vi "SSFG_sharp.vi"() -> ()   [LabVIEW 2014]
uses:
  SSFG_States.ctl
  <vilib>/Utility/error.llb/DialogType.ctl
  <vilib>/DAQmx/read.llb/DAQmx Read (Analog Wfm 1Chan NSamp).vi
  <vilib>/DAQmx/write.llb/DAQmx Write (Analog Wfm 1Chan NSamp).vi
  <vilib>/DAQmx/create/channels.llb/DAQmx Create Channel (AO-Voltage-Basic).vi
  <vilib>/DAQmx/create/channels.llb/DAQmx Create Channel (AI-Voltage-Basic).vi
  <vilib>/DAQmx/configure/timing.llb/DAQmx Timing (Sample Clock).vi
  <vilib>/DAQmx/miscellaneous.llb/DAQmx Fill In Error Info.vi
  <vilib>/measure/mascope.llb/Cycle Average and RMS 1 chan.vi
  <resource>/objmgr/daqmx.rc
  <vilib>/measure/NI_MABase.lvlib
  <vilib>/measure/NI_MAPro.lvlib
panel:
  in  "Physical Channel 2":tag="Dev1/ai0" caption="Physical Channel"
  in  "Sample Rate":dbl=10000.0 caption="Sample Rate (Hz)" format="%0.2f"
  out "Measurement":waveform(dbl)(graph)
  in  "stop 2":bool caption="stop"
  in  "Samples to Read":i32=1000
  out "cycle RMS":dbl format="%.2g"
  out "Numeric":i32
  out "Buffer Space":u32
  out "Iterations":i32
  in  "Attenuation":dbl
  in  "Number of Samples/Cycle":dbl
  out "Generation":waveform(dbl)(graph)
  in  "stop":bool
  in  "Power Signal Parameters":T1={"Waveform Type"=0, "Amplitude"=1.0, "Frequency"=17.0} {"Frequency" format="%0.2p"; "Waveform Type" items=["Sine Wave", "Triangle Wave", "Square Wave", "Sawtooth Wave"]}
  out "Flicker":bool
  out "Swell":bool
  out "Sag":bool
  in  "Stop":bool
  in  "Update Rate":dbl=1000.0 format="%0.2f"
  in  "Generation":tag
  in  "Flicker":T2
  in  "Swell":cluster{"Swell_Time (sec)":dbl, "Swell":bool}
  in  "Sag":cluster{"Sag_Time (sec)":dbl, "Sag":bool}
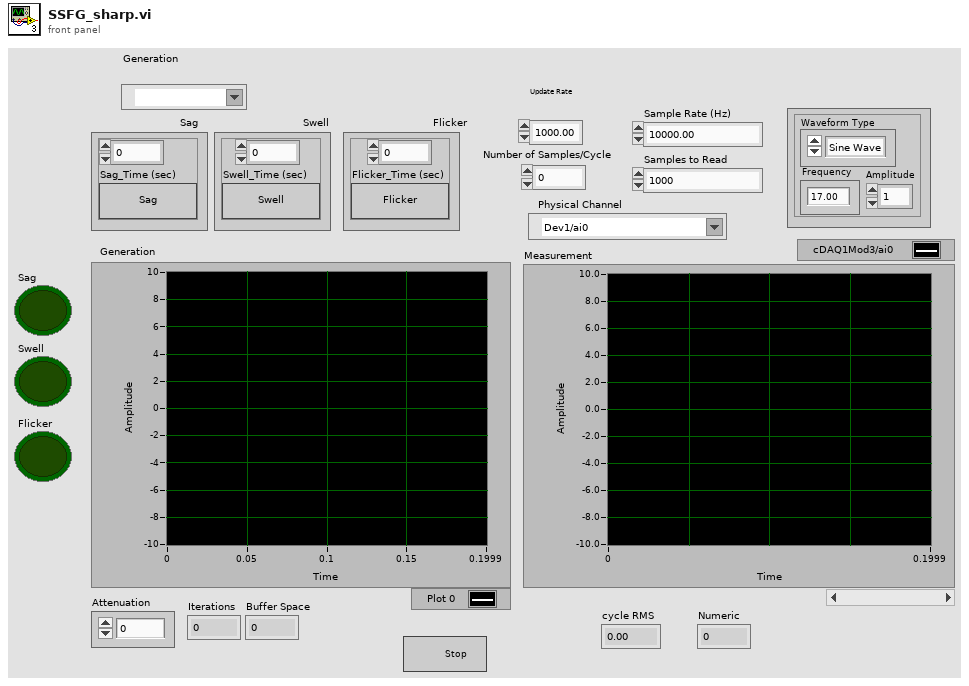
[diagram p1: front panel]
types:
  T1 = cluster{"Waveform Type":u16, "Amplitude":dbl, "Frequency":dbl}
  T2 = cluster{"Flicker_Time (sec)":dbl, "Flicker":bool}
  T3 = typedef "DialogType.ctl" = u16
  T4 = typedef "SSFG_States.ctl" = cluster{"State":string, "Disturbance_Time (sec)":dbl}
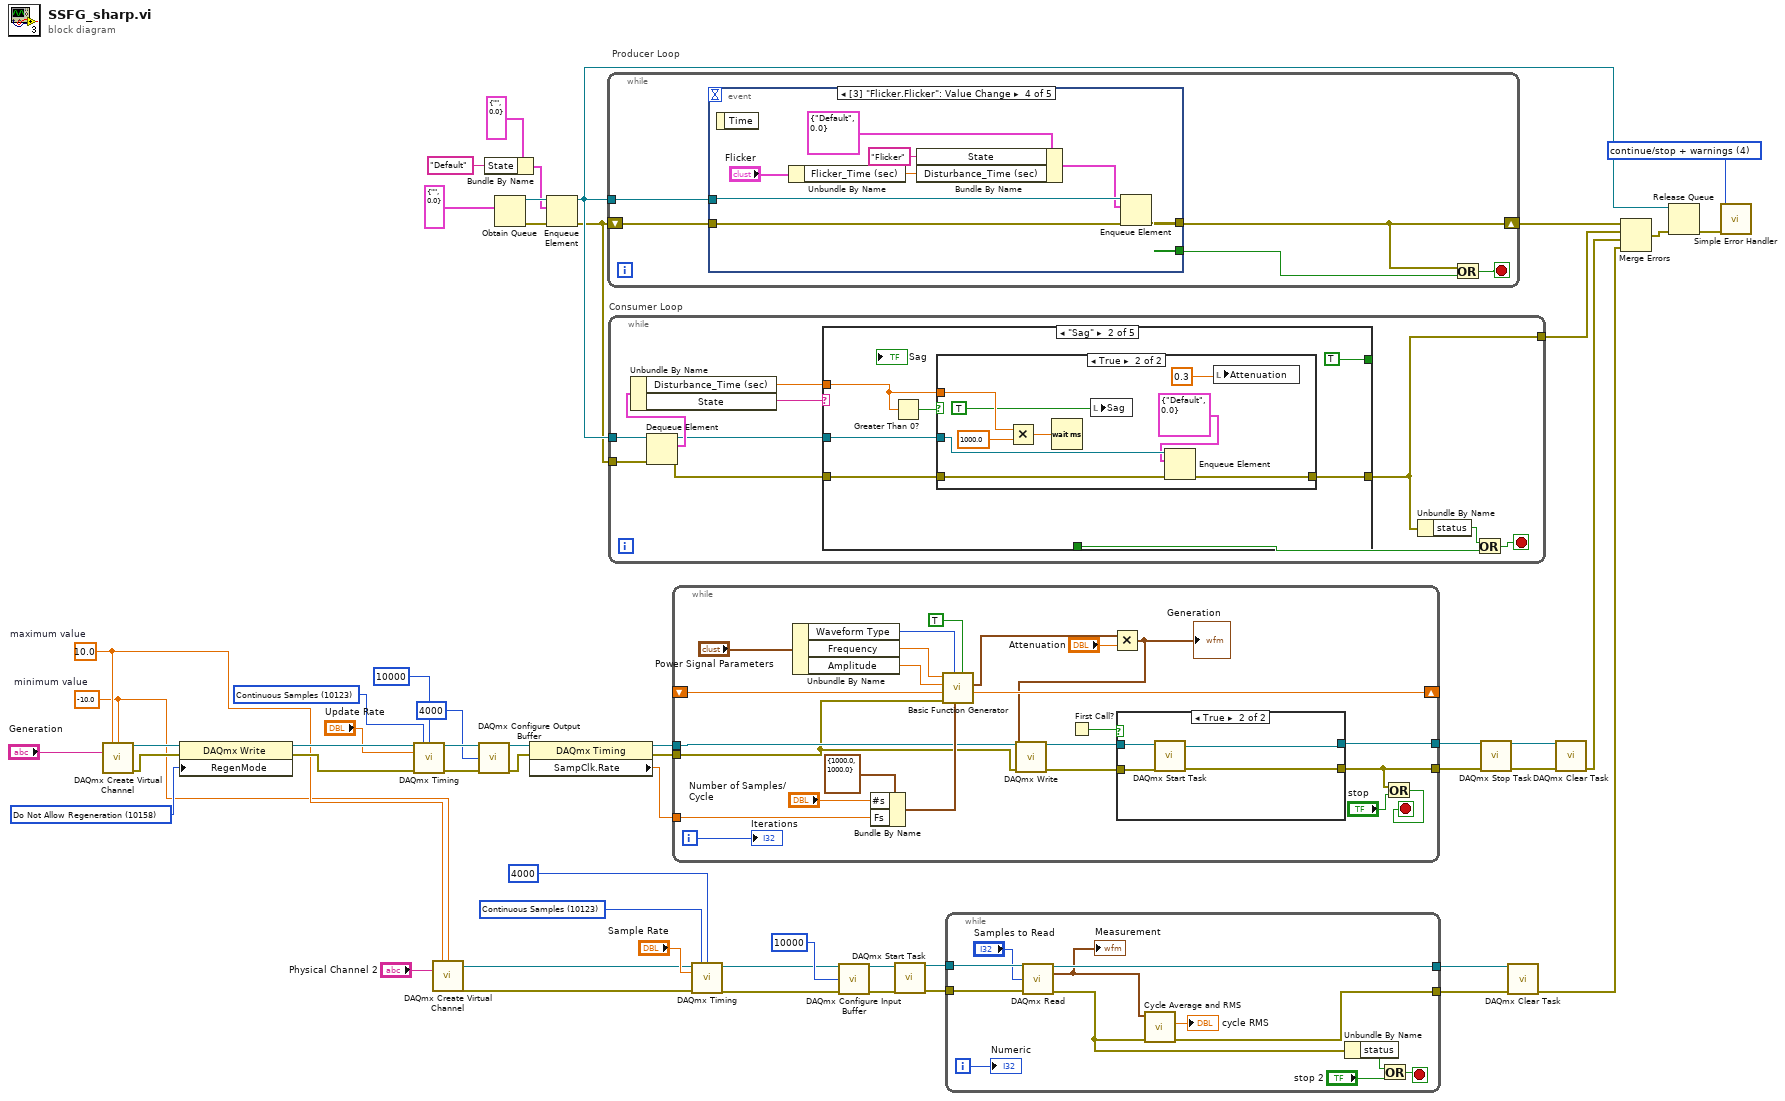
[diagram p0: block diagram]
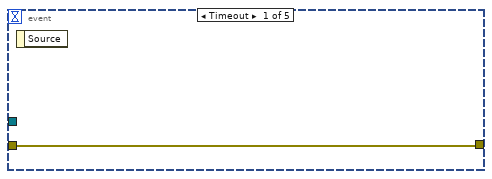
[diagram p2: hidden frame]
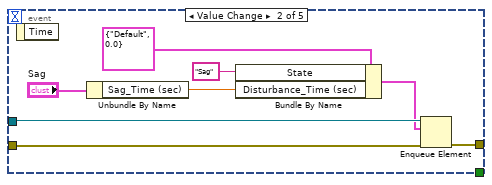
[diagram p3: hidden frame]
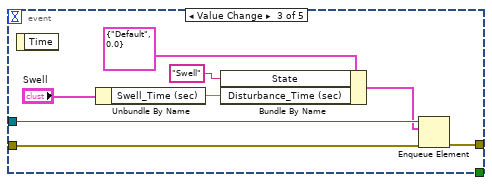
[diagram p4: hidden frame]
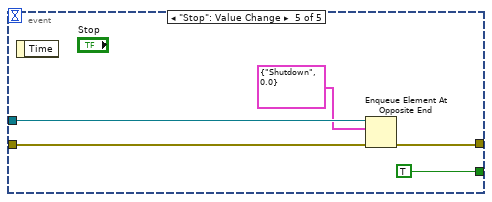
[diagram p5: hidden frame]
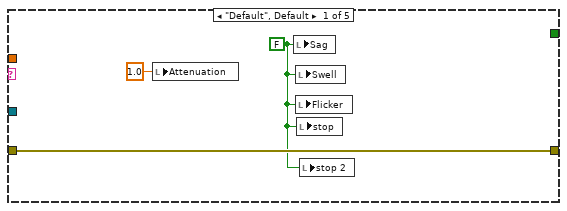
[diagram p6: hidden frame]
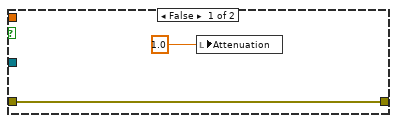
[diagram p7: hidden frame]
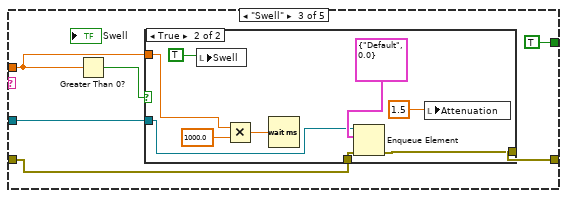
[diagram p8: hidden frame]
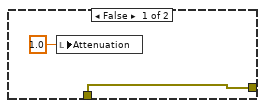
[diagram p9: hidden frame]
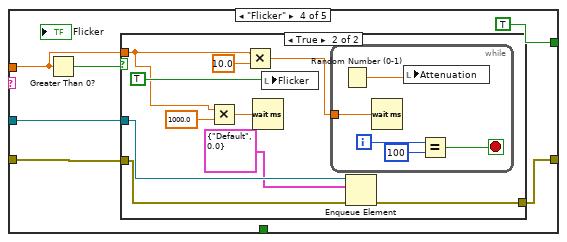
[diagram p10: hidden frame]
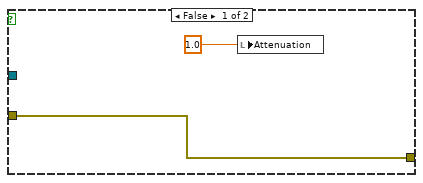
[diagram p11: hidden frame]
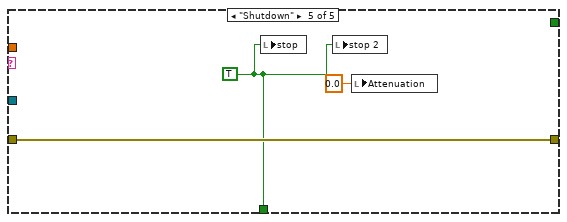
[diagram p12: hidden frame]
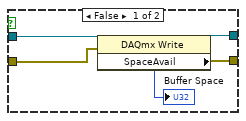
[diagram p13: hidden frame]
diagram:
  w1 = T3 4 items=["no dialog", "OK message", "continue or stop message", "OK message + warnings", "continue/stop + warnings"] ("type of dialog (OK msg:1)")
  w13 = 10123 items=["Finite Samples"=10178, "Continuous Samples"=10123] ("sample mode")
  w6 = 10.0  # maximum value
  w5 = -10.0  # minimum value
  w47 = 10123 items=["Finite Samples"=10178, "Continuous Samples"=10123, "Hardware Timed Single Point"=12522] ("sample mode")
  w48 = 10158 items=["Allow Regeneration"=10097, "Do Not Allow Regeneration"=10158] ("RegenMode")
  n1 = call-poly <vilib>:"DAQmx Create Virtual Channel.vi"("maximum value"=w6, "minimum value"=w5, "physical channels"="Generation") -> ("task out"=w52:refnum<k21>, "error out"=w50:errorcluster)  [unwired: 11 in]
  n2 = property class="DAQmx Write"(reference=w52, error in=w50, "RegenMode"=w48) -> (reference out=w51:refnum<k21>, error out=w49:errorcluster)
  n3 = call-poly <vilib>:"DAQmx Timing.vi"("task/channels in"=w51, "sample mode"=w47, "samples per channel"=10000, "rate"="Update Rate", "error in"=w49) -> ("task out"=w25:refnum<k21>, "error out"=w23:errorcluster)  [unwired: 9 in]
  n4 = call-poly <vilib>:"DAQmx Create Virtual Channel.vi"("maximum value"=w6, "minimum value"=w5, "physical channels"="Physical Channel 2") -> ("task out"=w9:refnum<k21>, "error out"=w7:errorcluster)  [unwired: 11 in]
  n5 = call <vilib>:"DAQmx Configure Output Buffer.vi"("task/channels in"=w25, "buffer size (in samples per channel)"=u32 4000, "error in"=w23) -> ("task out"=w24:refnum<k21>, "error out"=w22:errorcluster)  [unwired: 11 in]
  n6 = Bundle By Name(cluster=T4 {"State"="", "Disturbance_Time (sec)"=0.0}, "State"="Default") -> (w31:T4)
  n7 = Obtain Queue(element data type=T4 {"State"="", "Disturbance_Time (sec)"=0.0}) -> (queue out=w35:refnum<queue>, error out=w34:errorcluster)  [unwired: 4 in, 1 out]
  n8 = property class="DAQmx Timing"(reference=w24, error in=w22) -> (reference out=w43:refnum<k21>, error out=w44:errorcluster, "SampClk.Rate"=w42:dbl)
  n9 = Enqueue Element(queue=w35, element=w31, error in (no error)=w34) -> (queue out=w29:refnum<queue>, error out=w28:errorcluster)  [unwired: 1 in, 1 out]
  n10 = while "Producer Loop" {
    tunnel: w29 -> [w57]
    shift-right: [w55] -> w37
    shift-left: w28 -> [w56]
    stop <- w58 stop-if-true
    n11 = event shown="[3] \"Flicker.Flicker\": Value Change" {
      selector: _ -> [_ _ _ _ _]
      dyn-events: _ -> [_ _ _ _ _]
      timeout: _ -> [_ _ _ _ _]
      tunnel: w57 -> [_ w67 w75 w83 w88]
      tunnel: w56 -> [w59 w66 w74 w82 w87]
      tunnel: [w59 w65 w73 w81 w86] -> w55
      tunnel: [_ _ _ _ TRUE] -> w54
      event Timeout {
        n12 = event-data() -> ()  [unwired: 1 in, 1 out]
      }
      event "Sag.Sag": Value Change {
        n13 = event-data() -> ()  [unwired: 1 in, 1 out]
        n14 = Unbundle By Name("Sag") -> ("Sag_Time (sec)"=w62:dbl)
        n15 = Bundle By Name(cluster=T4 {"State"="Default", "Disturbance_Time (sec)"=0.0}, "State"="Sag", "Disturbance_Time (sec)"=w62) -> (w61:T4)
        n16 = Enqueue Element(queue=w67, element=w61, error in (no error)=w66) -> (error out=w65:errorcluster)  [unwired: 1 in, 2 out]
      }
      event "Swell.Swell": Value Change {
        n17 = event-data() -> ()  [unwired: 1 in, 1 out]
        n18 = Unbundle By Name("Swell") -> ("Swell_Time (sec)"=w71:dbl)
        n19 = Bundle By Name(cluster=T4 {"State"="Default", "Disturbance_Time (sec)"=0.0}, "State"="Swell", "Disturbance_Time (sec)"=w71) -> (w69:T4)
        n20 = Enqueue Element(queue=w75, element=w69, error in (no error)=w74) -> (error out=w73:errorcluster)  [unwired: 1 in, 2 out]
      }
      event "Flicker.Flicker": Value Change {
        n21 = event-data() -> ()  [unwired: 1 in, 1 out]
        n22 = Unbundle By Name("Flicker") -> ("Flicker_Time (sec)"=w78:dbl)
        n23 = Bundle By Name(cluster=T4 {"State"="Default", "Disturbance_Time (sec)"=0.0}, "State"="Flicker", "Disturbance_Time (sec)"=w78) -> (w77:T4)
        n24 = Enqueue Element(queue=w83, element=w77, error in (no error)=w82) -> (error out=w81:errorcluster)  [unwired: 1 in, 2 out]
      }
      event "Stop": Value Change {
        n25 = event-data() -> ()  [unwired: 1 in, 1 out]
        n26 = Enqueue Element At Opposite End(queue=w88, element=T4 {"State"="Shutdown", "Disturbance_Time (sec)"=0.0}, error in (no error)=w87) -> (error out=w86:errorcluster)  [unwired: 1 in, 2 out]
      }
    }
    n27 = Or(x=w55, y=w54) -> (x .or. y?=w58:bool)
  }
  n28 = while "Consumer Loop" {
    tunnel: [w92] -> w27
    tunnel: w29 -> [w97]
    tunnel: w28 -> [w96]
    stop <- w99 stop-if-true
    n29 = Dequeue Element(queue=w97, error in (no error)=w96) -> (queue out=w91:refnum<queue>, element=w95:T4, error out=w90:errorcluster)  [unwired: 1 in, 1 out]
    n30 = Unbundle By Name(w95) -> ("Disturbance_Time (sec)"=w89:dbl, "State"=w94:string)
    n31 = case shown="\"Sag\"" w94 {
      tunnel: [_ _ _ _ w160] -> w93
      tunnel: w90 -> [w102 w105 w123 w140 w161]
      tunnel: [w102 w106 w122 w139 w161] -> w92
      tunnel: w91 -> [_ w104 w121 w138 _]
      tunnel: w89 -> [_ w107 w124 w141 _]
      tunnel: [_ TRUE TRUE TRUE _] -> _
      frame "Default", Default {
        w100 = FALSE ("Sag")
        n32 = local write "Attenuation"(1.0 ("Attenuation")) -> ()
        n33 = local write "Sag"(w100) -> ()
        n34 = local write "Swell"(w100) -> ()
        n35 = local write "Flicker"(w100) -> ()
        n36 = local write "stop"(w100) -> ()
        n37 = local write "stop 2"(w100) -> ()
      }
      frame "Sag" {
        n38 = Greater Than 0?(x=w107) -> (x > 0?=w108:bool)
        n39 = case shown="True" w108 {
          tunnel: w107 -> [_ w113]
          tunnel: [w109 w118] -> w106
          tunnel: w105 -> [w109 w117]
          tunnel: w104 -> [_ w116]
          frame False {
            n40 = local write "Attenuation"(1.0 ("y")) -> ()
          }
          frame True {
            n41 = Multiply(x=w113, y=1000.0) -> (x*y=w114:dbl)
            n42 = Wait (ms)(milliseconds to wait=w114) -> ()  [unwired: 1 out]
            n43 = local write "Sag"(TRUE ("Auto Reset")) -> ()
            n44 = Enqueue Element(queue=w116, element=T4 {"State"="Default", "Disturbance_Time (sec)"=0.0}, error in (no error)=w117) -> (error out=w118:errorcluster)  [unwired: 1 in, 2 out]
            n45 = local write "Attenuation"(0.3 ("y")) -> ()
          }
        }
      }
      frame "Swell" {
        n46 = Greater Than 0?(x=w124) -> (x > 0?=w125:bool)
        n47 = case shown="True" w125 {
          tunnel: w124 -> [_ w131]
          tunnel: w123 -> [w126 w135]
          tunnel: [w126 w134] -> w122
          tunnel: w121 -> [_ w129]
          frame False {
            n48 = local write "Attenuation"(1.0 ("y")) -> ()
          }
          frame True {
            n49 = local write "Swell"(TRUE ("Auto Reset")) -> ()
            n50 = Multiply(x=w131, y=1000.0) -> (x*y=w133:dbl)
            n51 = Wait (ms)(milliseconds to wait=w133) -> ()  [unwired: 1 out]
            n52 = Enqueue Element(queue=w129, element=T4 {"State"="Default", "Disturbance_Time (sec)"=0.0}, error in (no error)=w135) -> (error out=w134:errorcluster)  [unwired: 1 in, 2 out]
            n53 = local write "Attenuation"(1.5 ("y")) -> ()
          }
        }
      }
      frame "Flicker" {
        n54 = Greater Than 0?(x=w141) -> (x > 0?=w142:bool)
        n55 = case shown="True" w142 {
          tunnel: w141 -> [_ w146]
          tunnel: w140 -> [w143 w154]
          tunnel: [w143 w153] -> w139
          tunnel: w138 -> [_ w152]
          frame False {
            n56 = local write "Attenuation"(1.0 ("y")) -> ()
          }
          frame True {
            n57 = Multiply(x=w146, y=1000.0) -> (x*y=w150:dbl)
            n58 = Multiply(x=w146, y=10.0) -> (x*y=w145:dbl)
            n59 = Wait (ms)(milliseconds to wait=w150) -> ()  [unwired: 1 out]
            n60 = local write "Flicker"(TRUE ("Auto Reset")) -> ()
            n61 = while {
              tunnel: w145 -> [w159]
              i -> [w157]
              stop <- w156 stop-if-true
              n62 = Random Number (0-1)() -> (number: 0 to 1=w158:dbl)
              n63 = Wait (ms)(milliseconds to wait=w159) -> ()  [unwired: 1 out]
              n64 = local write "Attenuation"(w158) -> ()
              n65 = Equal?(x=w157, y=100) -> (x = y?=w156:bool)
            }
            n66 = Enqueue Element(queue=w152, element=T4 {"State"="Default", "Disturbance_Time (sec)"=0.0}, error in (no error)=w154) -> (error out=w153:errorcluster)  [unwired: 1 in, 2 out]
          }
        }
      }
      frame "Shutdown" {
        w160 = TRUE
        n67 = local write "stop"(w160) -> ()
        n68 = local write "stop 2"(w160) -> ()
        n69 = local write "Attenuation"(0.0 ("Attenuation")) -> ()
      }
    }
    n70 = Unbundle By Name(w92) -> ("status"=w98:bool)
    n71 = Or(x=w98, y=w93) -> (x .or. y?=w99:bool)
  }
  n72 = while {
    tunnel: [w165] -> w41
    tunnel: [w177] -> w45
    tunnel: w43 -> [w167]
    tunnel: w44 -> [w166]
    tunnel: w42 -> [w175]
    shift-right: [w172] -> _
    shift-left: _ -> [w171]
    i -> [w168]
    stop <- w163 stop-if-true
    n73 = Unbundle By Name("Power Signal Parameters") -> ("Waveform Type"=w182:u16, "Frequency"=w181:dbl, "Amplitude"=w180:dbl)
    n74 = Bundle By Name(cluster=cluster{"Fs":dbl, "#s":dbl} {"Fs"=1000.0, "#s"=1000.0} ("sampling info"), "#s"="Number of Samples/Cycle", "Fs"=w175) -> (w176:cluster{"Fs":dbl, "#s":dbl})
    n75 = call <vilib>:"Basic Function Generator.vi"("reset signal"=TRUE, "sampling info"=w176, "signal type"=w182, "error in (no error)"=w166, "phase"=w171, "amplitude"=w180, "frequency"=w181) -> ("phase out"=w172:dbl, "signal out"=w173:waveform(dbl))  [unwired: 2 in, 1 out]
    n76 = First Call?() -> (First Call?: T/F=w183:bool)
    n77 = Multiply(x=w173, y="Attenuation") -> (x*y=w170:waveform(dbl))
    "Generation" <- w170
    n78 = call-poly <vilib>:"DAQmx Write.vi"("task/channels in"=w167, "data"=w170, "error in"=w166) -> ("task out"=w185:refnum<k21>, "error out"=w184:errorcluster)  [unwired: 10 in, 1 out]
    n79 = case shown="True" w183 {
      tunnel: w185 -> [w189 w195]
      tunnel: w184 -> [w188 w194]
      tunnel: [w190 w193] -> w177
      tunnel: [w191 w192] -> w165
      frame False {
        n80 = property class="DAQmx Write"(reference=w189, error in=w188) -> (reference out=w190:refnum<k21>, error out=w191:errorcluster, "SpaceAvail"=→"Buffer Space":u32)
      }
      frame True {
        n81 = call <vilib>:"DAQmx Start Task.vi"("task/channels in"=w195, "error in"=w194) -> ("task out"=w193:refnum<k21>, "error out"=w192:errorcluster)  [unwired: 12 in]
      }
    }
    n82 = Or(x=w165, y="stop") -> (x .or. y?=w163:bool)
    "Iterations" <- w168
  }
  n83 = call-poly <vilib>:"DAQmx Timing.vi"("task/channels in"=w9, "sample mode"=w13, "samples per channel"=u32 4000 ("buffer size (in samples per channel)"), "rate"="Sample Rate", "error in"=w7) -> ("task out"=w16:refnum<k21>, "error out"=w17:errorcluster)  [unwired: 9 in]
  n84 = call <vilib>:"DAQmx Configure Input Buffer.vi"("task/channels in"=w16, "buffer size (in samples per channel)"=u32 10000, "error in"=w17) -> ("task out"=w19:refnum<k21>, "error out"=w18:errorcluster)  [unwired: 11 in]
  n85 = call <vilib>:"DAQmx Start Task.vi"("task/channels in"=w19, "error in"=w18) -> ("task out"=w10:refnum<k21>, "error out"=w8:errorcluster)  [unwired: 12 in]
  n86 = while {
    tunnel: w8 -> [w207]
    tunnel: w10 -> [w206]
    tunnel: [w205] -> w11
    tunnel: [w199] -> w14
    i -> [w201]
    stop <- w196 stop-if-true
    n87 = call-poly <vilib>:"DAQmx Read.vi"("task/channels in"=w206, "number of samples per channel"="Samples to Read", "error in"=w207) -> ("task out"=w205:refnum<k21>, "data"=w203:waveform(dbl), "error out"=w200:errorcluster)  [unwired: 10 in]
    "Measurement" <- w203
    n88 = call-poly <vilib>:"Cycle Average and RMS.vi"("error in (no error)"=w200, "signal in"=w203) -> ("error out"=w199:errorcluster, "cycle RMS"=→"cycle RMS":dbl)  [unwired: 6 in, 2 out]
    n89 = Unbundle By Name(w200) -> ("status"=w197:bool)
    n90 = Or(x=w197, y="stop 2") -> (x .or. y?=w196:bool)
    "Numeric" <- w201
  }
  n91 = call <vilib>:"DAQmx Stop Task.vi"("task/channels in"=w45, "error in"=w41) -> ("task out"=w40:refnum<k21>, "error out"=w39:errorcluster)  [unwired: 12 in]
  n92 = call <vilib>:"DAQmx Clear Task.vi"("task in"=w11, "error in"=w14) -> ("error out"=w4:errorcluster)  [unwired: 13 in]
  n93 = call <vilib>:"DAQmx Clear Task.vi"("task in"=w40, "error in"=w39) -> ("error out"=w26:errorcluster)  [unwired: 13 in]
  n94 = Merge Errors(w37, w27, w26, w4) -> (w36:errorcluster)
  n95 = Release Queue(queue=w29, error in (no error)=w36) -> (error out=w38:errorcluster)  [unwired: 1 in, 2 out]
  n96 = call <vilib>:"Simple Error Handler.vi"("type of dialog (OK msg:1)"=w1, "error in (no error)"=w38) -> ()  [unwired: 3 in, 5 out]
